vi "Ex4ROIExample.vi"() -> ()   [LabVIEW 2010]
panel:
  in  "Exposure":dbl min=0.0 step=0.001 format="%.3f"
  in  "stop":bool
  in  "Store":bool
  out "error out":errorcluster
  in  "error in (no error)":errorcluster
  # "Ex4ROIExample - 4 corners of CCD"
  # "Description: This example shows\nhow to collect multiple ROIs for \nan image. It takes the 4 corners\nof the CCD camera"
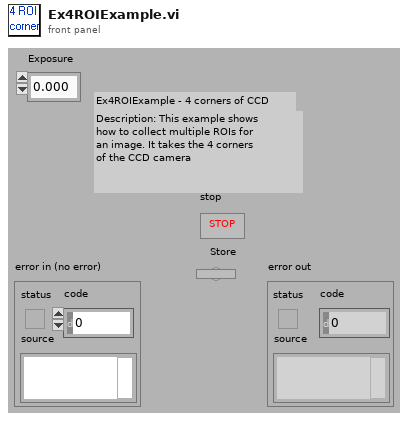
[diagram p1: front panel]
types:
  T1 = cluster{"Acquire Focus Mode, 3 is async which should be good for all cameras":i32, "Exposure":dbl, "Number of images":i32, "Software Accumulation":i32}
  T2 = cluster{"Camera Handle":u32, "Pulser Handle":u32, "File Handle":u32, "Display Handle":u32, "Image Handle":u32}
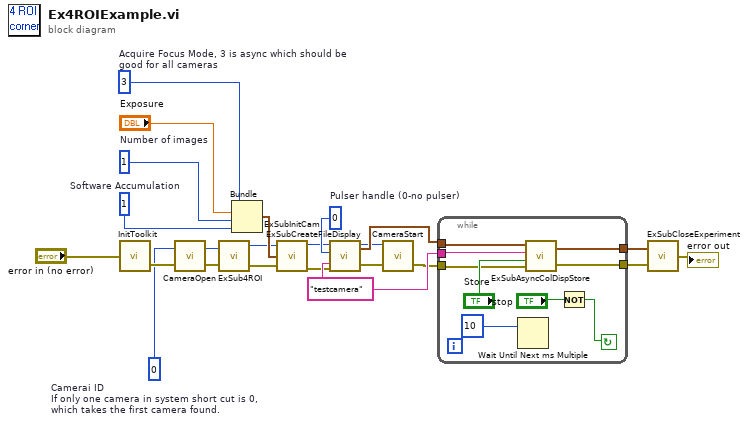
[diagram p0: block diagram]
diagram:
  w6 = 0  # Camerai ID If only one camera in system short cut is 0,  which takes the first camera found.
  w15 = 0  # Pulser handle (0-no pulser)
  w20 = 1  # Number of images
  w21 = 3  # Acquire Focus Mode, 3 is async which should be good for all cameras
  w19 = 1  # Software Accumulation
  w22 = "testcamera"
  n1 = call <userlib>:"InitToolkit.vi"("error in"="error in (no error)") -> ("error out"=w7:errorcluster)
  n2 = call <userlib>:"CameraOpen.vi"("error in"=w7, "Camera Device ID"=w6) -> ("error out"=w4:errorcluster, "Camera Handle"=w5:u32)
  n3 = call "ExSub4ROI.vi"("error in (no error)"=w4, "Camera Handle"=w5) -> ("error out"=w3:errorcluster, "Camera Handle"=w2:u32)
  n4 = Bundle("Acquire Focus Mode, 3 is async which should be good for all cameras"=w21, "Exposure"="Exposure", "Number of images"=w20, "Software Accumulation"=w19) -> (w17:T1)  [unwired: 1 in]
  n5 = call "ExSubInitCam.vi"("error in (no error)"=w3, "Camera Information"=w17, "Camera Handle"=w2) -> ("error out"=w16:errorcluster, "Camera Handle"=w1:u32)
  n6 = call "ExSubCreateFileDisplay.vi"("error in (no error)"=w16, "File and Display Name"=w22, "Pulser Handle"=w15, "Camera Handle"=w1) -> ("error out"=w14:errorcluster, "Handles Out"=w13:T2)
  n7 = call <userlib>:"CameraStart.vi"("error in"=w14, "Camera Handle"=w1) -> ("error out"=w12:errorcluster)  [unwired: 1 out]
  n8 = while {
    tunnel: w13 -> [w29]
    tunnel: w12 -> [w27]
    tunnel: w22 -> [w28]
    tunnel: [w25] -> w10
    tunnel: [w26] -> w11
    stop <- w24 continue-if-true
    n9 = Wait Until Next ms Multiple(millisecond multiple=10) -> ()  [unwired: 1 out]
    n10 = call "ExSubAsyncColDispStore.vi"("error in (no error)"=w27, "Store Data"="Store", "Display Title"=w28, "Handle Cluster"=w29) -> ("error out"=w25:errorcluster, "Handle Cluster Out"=w26:T2)
    n11 = Not(x="stop") -> (.not. x?=w24:bool)
  }
  n12 = call "ExSubCloseExperiment.vi"("error in (no error)"=w10, "Handles In"=w11) -> ("error out"=→"error out":errorcluster)
